vi "TWM Client Cmd Start.vi"(7 "end of packet key":string="TWM:command:EndOfPacket", 8 "error in":errorcluster, 11 "handle":i32) -> (0 "error out":errorcluster, 3 "handle out":i32)   [LabVIEW 2013]
doc: "Write Start command packet to TWM server."
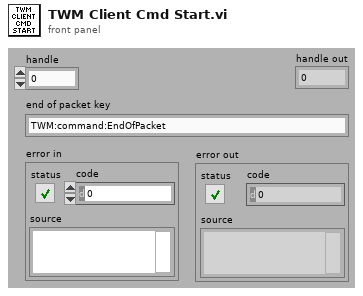
[diagram p1: front panel]
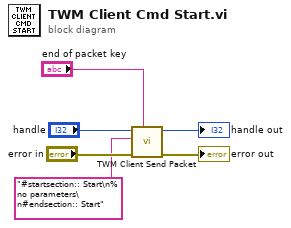
[diagram p0: block diagram]
diagram:
  n1 = call "TWM Client Send Packet.vi"("end of packet key"="end of packet key", "error in"="error in", "command string"="#startsection:: Start\n% no parameters\n#endsection:: Start", "handle"="handle") -> ("error out"=→"error out":errorcluster, "handle out"=→"handle out":i32)  [unwired: 6 in]
